vi "close.vi"(8 "error in":errorcluster, 11 "Profibus Module runtime in":refnum<class "Profibus Module runtime.lvclass">) -> (0 "error out":errorcluster)   [LabVIEW 2013, in "Profibus Module runtime.lvclass"]
doc: "Provides an interface for terminating a module instance. While this interface performs no operations, a child should close and deallocate any open references or memory."
uses:
  Profibus Module runtime.lvclass
  <vilib>/addons/Comsoft.lib/cRIO PBMS/CS_cRIO-PB_DP-Master_FPGA-Reference.ctl
  <vilib>/rvi/interface/nirviCloseFPGA/nirviCloseFPGA.xnode
  <vilib>/FPGAPlugInAG/Dynamic/niLvFpga_Close_Dynamic.vi
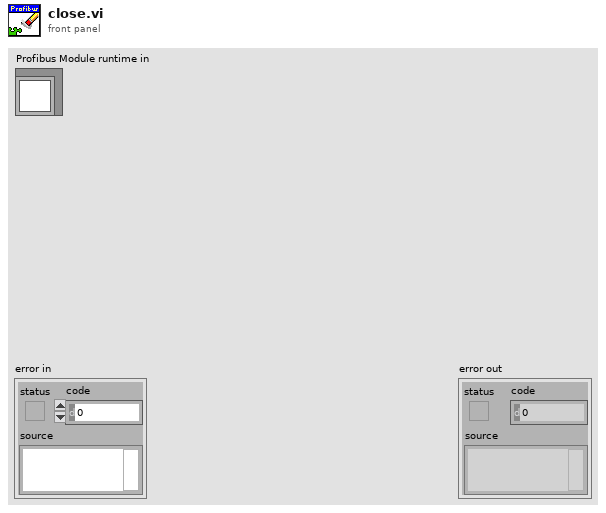
[diagram p1: front panel]
types:
  T1 = typedef "CS_cRIO-PB_DP-Master_FPGA-Reference.ctl" = refnum<k20>
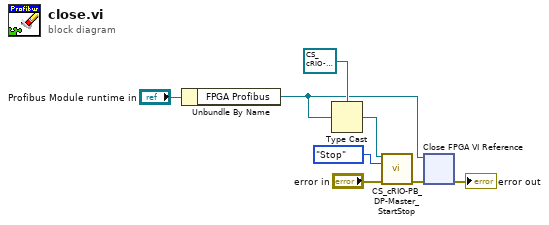
[diagram p0: block diagram]
diagram:
  n1 = Unbundle By Name("Profibus Module runtime in") -> ("FPGA Profibus"=w1:refnum<k20>)
  n2 = Type Cast(type=T1 refnum ("FPGA VI Reference out"), x=w1) -> (*(type *) &x=w2:T1)
  n3 = call <vilib>:"CS_cRIO-PB_DP-Master_StartStop.vi"("FPGA VI Reference"=w2, "DP-Master"=enum16{"Start", "Stop"}."Stop", "Error"="error in") -> ("Error out"=w6:errorcluster)  [unwired: 10 in, 2 out]
  n4 = xnode "Close FPGA VI Reference"("FPGA VI Reference In"=w1, "error in"=w6) -> ("error out"=→"error out":errorcluster)
